vi "Evaluate Answer.vi"(0 "Candidate ID":string, 5 "Question_ID":string, 7 "Solution Path":path, 11 "error in (no error)":errorcluster) -> (4 "Result":T1, 15 "error out":errorcluster)   [LabVIEW 2014, in "Coding Platform.lvlib"]
uses:
  Coding Platform.lvlib
  Typedefs/User Event Operations.ctl
  Datatypes/Evaluation Result.ctl
  Datatypes/Evaluate Result.ctl
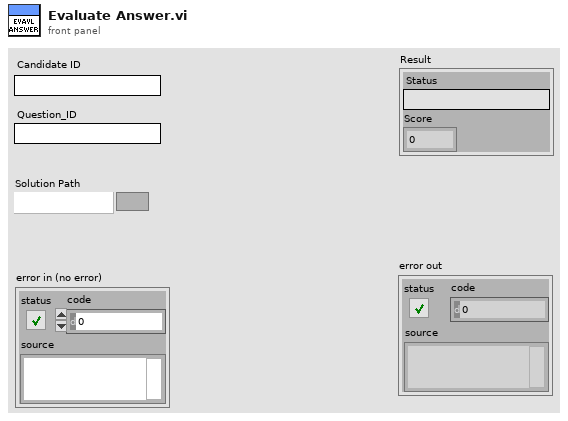
[diagram p1: front panel]
types:
  T1 = typedef "Coding Platform.lvlib/Evaluation Result.ctl" = cluster{"Status":string, "Score":u64}
  T2 = typedef "Coding Platform.lvlib/Evaluate Result.ctl" = cluster{"Candidate_ID":string, "notifier":refnum<notifier>, "Question_ID":string, "Solution Path":path}
  T3 = typedef "Coding Platform.lvlib/User Event Operations.ctl" = enum16{"Create", "Genereate", "Destroy", "Get Reference"}
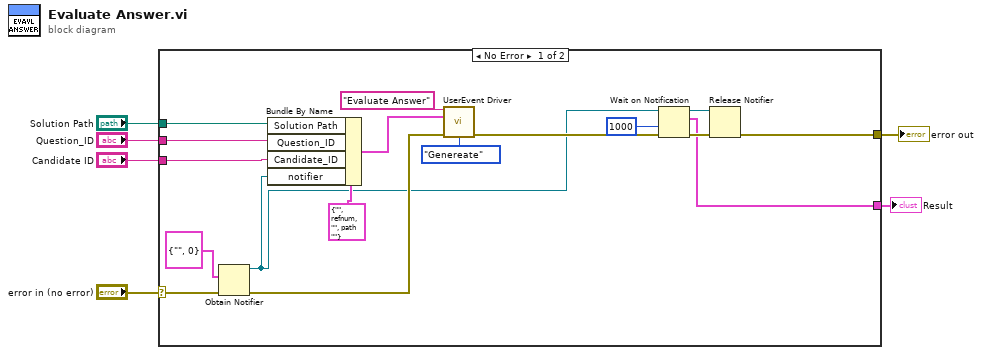
[diagram p0: block diagram]
diagram:
  n1 = case shown="No Error" "error in (no error)" {
    selector: "error in (no error)" -> [w11 w24]
    tunnel: [w15 w24] -> w6
    tunnel: "Candidate ID" -> [w18 _]
    tunnel: [w13 _] -> w1
    tunnel: "Question_ID" -> [w8 _]
    tunnel: "Solution Path" -> [w7 _]
    frame No Error {
      n2 = Obtain Notifier(notification data type=T1 {"Status"="", "Score"=0}, error in (no error)=w11) -> (notifier out=w9:refnum<notifier>, error out=w12:errorcluster)  [unwired: 2 in, 1 out]
      n3 = Bundle By Name(cluster=T2 {"Candidate_ID"="", "notifier"=refnum, "Question_ID"="", "Solution Path"=path ""} ("Login"), "Solution Path"=w7, "Question_ID"=w8, "Candidate_ID"=w18, "notifier"=w9) -> (w19:T2)
      n4 = call "UserEvent Driver.vi"("Message"="Evaluate Answer", "Data"=w19, "error in (no error)"=w12, "Operations(Get Reference)"=User_Event_Operations."Genereate") -> ("error out"=w23:errorcluster)  [unwired: 10 in, 1 out]
      n5 = Wait on Notification(notifier=w9, timeout in ms (-1)=1000, error in (no error)=w23) -> (notifier out=w14:refnum<notifier>, notification=w13:T1, error out=w17:errorcluster)  [unwired: 1 in, 1 out]
      n6 = Release Notifier(notifier=w14, error in (no error)=w17) -> (error out=w15:errorcluster)  [unwired: 1 in, 2 out]
    }
    frame Error {
    }
  }
  "error out" <- w6
  "Result" <- w1
